vi "ErrorDialog.vi"(8 "error in":errorcluster) -> (0 "error out":errorcluster)   [LabVIEW 2009]
panel:
  out "Message":string
  in  "OK":bool
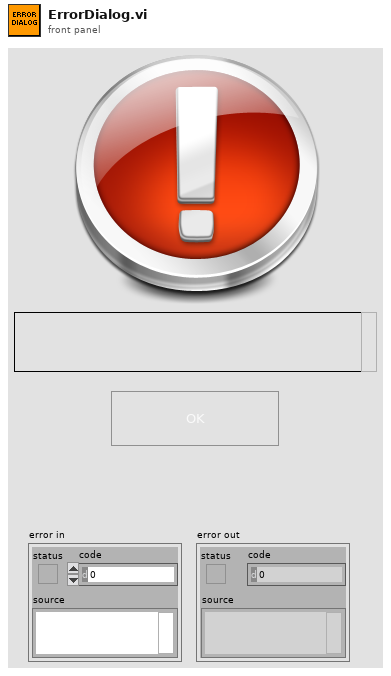
[diagram p1: front panel]
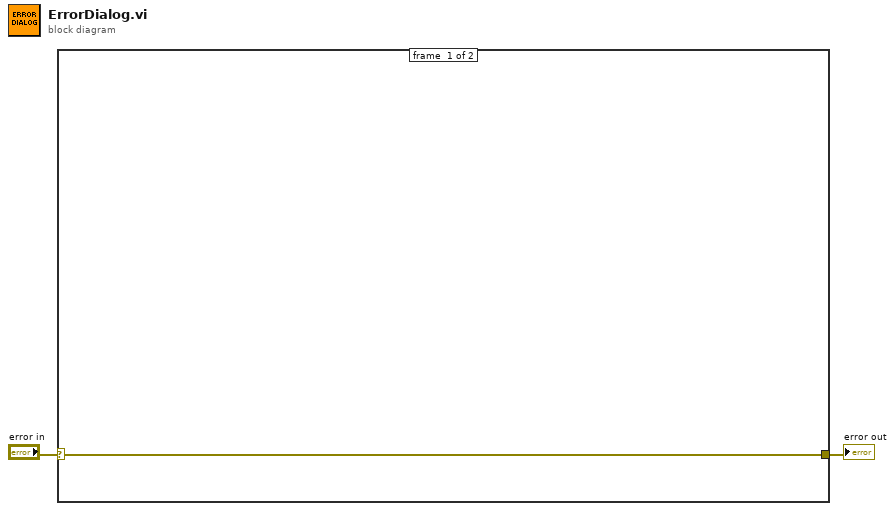
[diagram p0: block diagram]
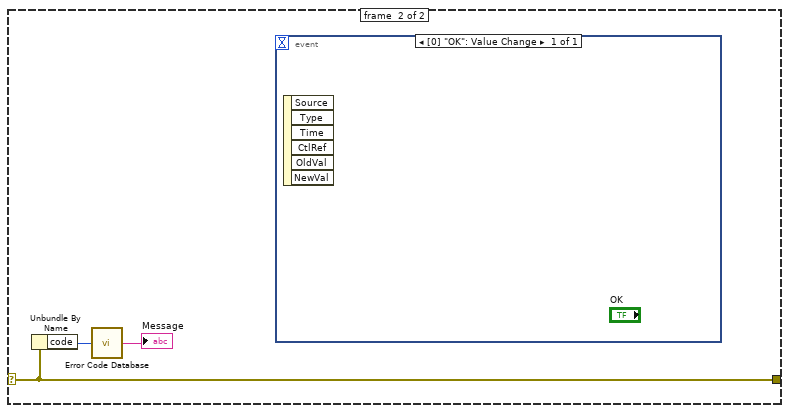
[diagram p2: hidden frame]
diagram:
  n1 = case shown="Error" "error in" {
    selector: "error in" -> [w3 w6]
    tunnel: [w3 w6] -> w1
    frame #0 {
    }
    frame #1 {
      n2 = Unbundle By Name(w6) -> ("code"=w5:i32)
      n3 = call <vilib>:"Error Code Database.vi"("Error Code"=w5) -> ("Error Text"=→"Message":string)
      n4 = event shown="[0] \"OK\": Value Change" {
        selector: _ -> [_]
        dyn-events: _ -> [_]
        timeout: _ -> [_]
        event [0] "OK": Value Change {
          n5 = event-data() -> ()  [unwired: 7 out]
        }
      }
    }
  }
  "error out" <- w1
